vi "CountVectorizer.vi"(8 "error in":errorcluster caption="entrée d'erreur", 11 "CountVectorizer":T1={"encoding"="utf-8", "decode_error"="strict", "strip_accents"="None", "lowercase"=TRUE, "preprocessor"="None", "tokenizer"="None", "stop_words"={"Type"="None", "list"=[]}, "token_pattern"="(?u)\\b\\w\\w+\\b", "ngram_range"={"min_n"=1, "max_n"=1}, "analyzer"="word", "max_df"=1.0, "min_df"=1.0, "max_features"=-1, "vocabulary"={"Clé"=["None"], "Valeur"=[]}, "binary"=FALSE, "dtype"="int"} {"max_features" min=-1; "min_df" min=0.0 max=1.0; "max_df" min=0.0 max=1.0}) -> (0 "error out":errorcluster caption="sortie d'erreur", 3 "CountVectorizer.lvclass":refnum<class "CountVectorizer.lvclass">)   [LabVIEW 2020]
doc: "Convert a collection of text documents to a matrix of token counts\n\nThis implementation produces a sparse representation of the counts using scipy.sparse.csr_matrix.\n\nIf you do not provide an a-priori dictionary and you do not use an analyzer that does some kind of feature selection then the number of features will be equal to the vocabulary size found by analyzing the data.\n\n\nParameters :\n\n- encoding : string, default=’utf-8’\nIf bytes or files are given to analyze, this encoding is used to decode.\n\n- decode_error : {‘strict’, ‘ignore’, ‘replace’}, default=’strict’\nInstruction on what to do if a byte sequence is given to analyze that contains characters not of the given encoding. By default, it is ‘strict’, meaning that a UnicodeDecodeError will be raised. Other values are ‘ignore’ and ‘replace’.\n\n- strip_accents : {‘ascii’, ‘unicode’}, default=None\nRemove accents and perform other character normalization during the preprocessing step. ‘ascii’ is a fast method that only works on characters that have an direct ASCII mapping. ‘unicode’ is a slightly slower method that works on any characters. None (default) does nothing.\n\n- lowercase : bool, default=True\nConvert all characters to lowercase before tokenizing.\n\n- preprocessor : callable, default=None\nOverride the preprocessing (string transformation) stage while preserving the tokenizing and n-grams generation steps. Only applies if analyzer is not callable.\n\n- tokenizer : callable, default=None\nOverride the string tokenization step while preserving the preprocessing and n-grams generation steps. Only applies if analyzer == 'word'.\n\n- stop_words : string {‘english’}, list, default=None\nIf ‘english’, a built-in stop word list for English is used. There are several known issues with ‘english’ and you should consider an alternative.\n\nIf a list, that list is assumed to contain stop words, all of which will be removed from the resulting tokens. Only applies if analyzer == 'word'.\n\nIf None, no stop words will be used. max_df can be set to a value in the range [0.7, 1.0) to automatically detect and filter stop words based on intra corpus document frequency of terms.\n\n- token_pattern : string\nRegular expression denoting what constitutes a “token”, only used if analyzer == 'word'. The default regexp select tokens of 2 or more alphanumeric characters (punctuation is completely ignored and always treated as a token separator).\n\n- ngram_range : tuple (min_n, max_n), default=(1, 1)\nThe lower and upper boundary of the range of n-values for different word n-grams or char n-grams to be extracted. All values of n such such that min_n <= n <= max_n will be used. For example an ngram_range of (1, 1) means only unigrams, (1, 2) means unigrams and bigrams, and (2, 2) means only bigrams. Only applies if analyzer is not callable.\n\n- analyzer : string, {‘word’, ‘char’, ‘char_wb’} or callable, default=’word’\nWhether the feature should be made of word n-gram or character n-grams. Option ‘char_wb’ creates character n-grams only from text inside word boundaries; n-grams at the edges of words are padded with space.\n\nIf a callable is passed it is used to extract the sequence of features out of the raw, unprocessed input.\n\n- max_df : float in range [0.0, 1.0] or int, default=1.0\nWhen building the vocabulary ignore terms that have a document frequency strictly higher than the given threshold (corpus-specific stop words). If float, the parameter represents a proportion of documents, integer absolute counts. This parameter is ignored if vocabulary is not None.\n\n- min_df : float in range [0.0, 1.0] or int, default=1\nWhen building the vocabulary ignore terms that have a document frequency strictly lower than the given threshold. This value is also called cut-off in the literature. If float, the parameter represents a proportion of documents, integer absolute counts. This parameter is ignored if vocabulary is not None.\n\n- max_features : int, default=None=-1\nIf not None, build a vocabulary that only consider the top max_features ordered by term frequency across the corpus.\n\nThis parameter is ignored if vocabulary is not None.\n\n- vocabulary : Mapping or iterable, default=None\nEither a Mapping (e.g., a dict) where keys are terms and values are indices in the feature matrix, or an iterable over terms. If not given, a vocabulary is determined from the input documents. Indices in the mapping should not be repeated and should not have any gap between 0 and the largest index.\n\n- binary : bool, default=False\nIf True, all non zero counts are set to 1. This is useful for discrete probabilistic models that model binary events rather than integer counts.\n\n- dtype : type, default=np.int64\nType of the matrix returned by fit_transform() or transform().\n\n\n\n\nMethods : \n\n- Decode the input into a string of unicode symbols. The decoding strategy depends on the vectorizer parameters.\n\nParameters : doc : str\n The string to decode.\n\nReturns : doc : str\n A string of unicode symbols.\n\n\n- Fit : Learn a vocabulary dictionary of all tokens in the raw documents.\n\nParameters : raw_documents : iterable\n An iterable which yields either str, unicode or file objects.\n\nReturns : String : OK\n\n- Fit Transform : Learn the vocabulary dictionary and return document-term matrix. This is equivalent to fit followed by transform, but more efficiently implemented.\n\nParameters : raw_documents : iterable\n An iterable which yields either str, unicode or file objects.\n\nReturns : X : array of shape (n_samples, n_features)\n Document-term matrix.\n\n- Get Feature Names : Array mapping from feature integer indices to feature name.\n\nReturns : feature_names : list\n A list of feature names.\n\n-Transform : Transform documents to document-term matrix. Extract token counts out of raw text documents using the vocabulary fitted with fit or the one provided to the constructor.\n\nParameters : raw_documents : iterable\n An iterable which yields either str, unicode or file objects.\n\nReturns : X : sparse matrix of shape (n_samples, n_features)\n Document-term matrix."
uses:
  CountVectorizer.lvclass
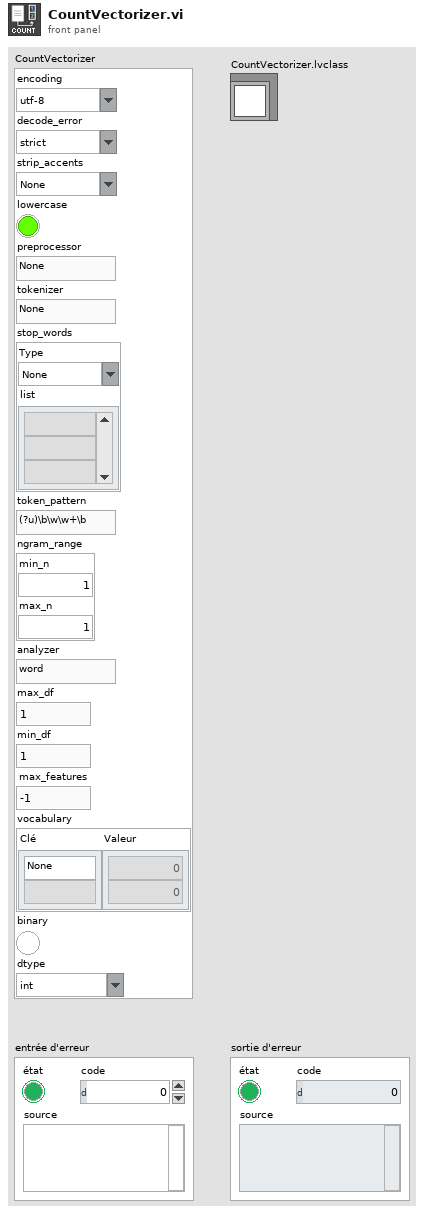
[diagram p1: front panel]
types:
  T1 = cluster{"encoding":string, "decode_error":string, "strip_accents":string, "lowercase":bool, "preprocessor":string, "tokenizer":string, "stop_words":cluster{"Type":string, "list":string[]}, "token_pattern":string, "ngram_range":cluster{"min_n":i32, "max_n":i32}, "analyzer":string, "max_df":dbl, "min_df":dbl, "max_features":i32, "vocabulary":cluster{"Clé":string[], "Valeur":i32[]}, "binary":bool, "dtype":string}
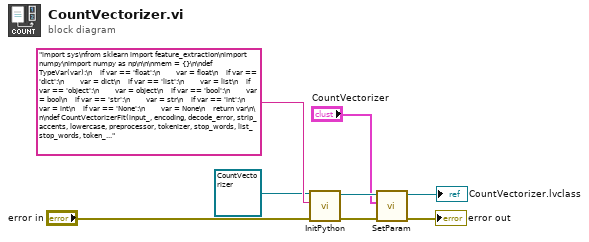
[diagram p0: block diagram]
diagram:
  n1 = call-dynamic "InitPython.vi"("error in (no error)"="error in", "Python Instruction"="import sys\nfrom sklearn import feature_extraction\nimport numpy\nimport numpy as np\n\n\nmem = {}\n\ndef TypeVar(var):\n    if var == 'float':\n        var = float\n    if var == 'dict':\n        var = dict\n    if var == 'list':\n        var = list\n    if var == 'object':\n        var = object\n    if var == 'bool':\n        var = bool\n    if var == 'str':\n        var = str\n    if var == 'int':\n        var = int\n    if var == 'None':\n        var = None\n    return var\n\n\ndef CountVectorizerFit(input_, encoding, decode_error, strip_accents, lowercase, preprocessor, tokenizer, stop_words, list_stop_words, token_pattern, min_n, max_n, analyzer, max_df, min_df, max_features, vocabulary, binary, dtype, X, doc):\n    X = eval(X)\n    dtype = TypeVar(dtype)\n    list_analyzer = ['word', 'char', 'char_wb']\n    if vocabulary == 'None':\n        vocabulary = None\n    else:\n        vocabulary = eval(vocabulary)\n    if tokenizer == 'None' or tokenizer == '':\n        tokenizer = None\n    else:\n        tokenizer = eval(tokenizer)\n    if preprocessor == 'None' or preprocessor == '':\n        preprocessor = None\n    else:\n        preprocessor = eval(preprocessor)\n    if strip_accents == 'None':\n        strip_accents = None\n    if stop_words == 'None':\n        stop_words = None\n    elif stop_words == 'list':\n        stop_words = list_stop_words\n    else: \n        pass\n    if max_features == -1:\n        max_features = None\n    if analyzer not in list_analyzer:\n        analyzer = eval(analyzer)  \n    try:\n        CountVectorizer = feature_extraction.text.CountVectorizer(input_, encoding, decode_error, strip_accents, lowercase, preprocessor, tokenizer, stop_words, token_pattern, (min_n, max_n), analyzer, max_df, min_df, max_features, vocabulary, binary, dtype).fit(X)\n        mem['FitCountVectorizer'] = CountVectorizer\n        return str('OK')\n    except:\n        erreur = sys.exc_info()\n        typerr = u\"%s\" % (erreur[0])\n        typerr = typerr[typerr.find(\"'\")+1:typerr.rfind(\"'\")]\n        msgerr = u\"%s\" % (erreur[1])\n        message = str('/!\\\\ {0} : {1}'. format(typerr,msgerr))\n        return message \n\ndef CountVectorizerFitTransform(input_, encoding, decode_error, strip_accents, lowercase, preprocessor, tokenizer, stop_words, list_stop_words, token_pattern, min_n, max_n, analyzer, max_df, min_df, max_features, vocabulary, binary, dtype, X, doc):\n    X = eval(X)\n    dtype = TypeVar(dtype)\n    list_analyzer = ['word', 'char', 'char_wb']\n    if vocabulary == 'None':\n        vocabulary = None\n    else:\n        vocabulary = eval(vocabulary)\n    if tokenizer == 'None' or tokenizer == '':\n        tokenizer = None\n    else:\n        tokenizer = eval(tokenizer)\n    if preprocessor == 'None' or preprocessor == '':\n        preprocessor = None\n    else:\n        preprocessor = eval(preprocessor)\n    if strip_accents == 'None':\n        strip_accents = None\n    if stop_words == 'None':\n        stop_words = None\n    elif stop_words == 'list':\n        stop_words = list_stop_words\n    else: \n        pass\n    if max_features == -1:\n        max_features = None\n    if analyzer not in list_analyzer:\n        analyzer = eval(analyzer)  \n    try:\n        CountVectorizer = feature_extraction.text.CountVectorizer(input_, encoding, decode_error, strip_accents, lowercase, preprocessor, tokenizer, stop_words, token_pattern, (min_n, max_n), analyzer, max_df, min_df, max_features, vocabulary, binary, dtype).fit_transform(X)\n        dtype = type(CountVectorizer)\n        if dtype == numpy.ndarray:\n            CountVectorizer = CountVectorizer.tolist()\n            return str(CountVectorizer)\n        else:\n            Mat = CountVectorizer.tocoo()\n            return str(list(zip(Mat.row, Mat.col, Mat.data)))\n    except:\n        erreur = sys.exc_info()\n        typerr = u\"%s\" % (erreur[0])\n        typerr = typerr[typerr.find(\"'\")+1:typerr.rfind(\"'\")]\n        msgerr = u\"%s\" % (erreur[1])\n        message = str('/!\\\\ {0} : {1}'. format(typerr,msgerr))\n        return message \n    \ndef CountVectorizerTransform(input_, encoding, decode_error, strip_accents, lowercase, preprocessor, tokenizer, stop_words, list_stop_words, token_pattern, min_n, max_n, analyzer, max_df, min_df, max_features, vocabulary, binary, dtype, X, doc):\n    X = eval(X)\n    dtype = TypeVar(dtype)\n    list_analyzer = ['word', 'char', 'char_wb']\n    if vocabulary == 'None':\n        vocabulary = None\n    else:\n        vocabulary = eval(vocabulary)\n    if tokenizer == 'None' or tokenizer == '':\n        tokenizer = None\n    else:\n        tokenizer = eval(tokenizer)\n    if preprocessor == 'None' or preprocessor == '':\n        preprocessor = None\n    else:\n        preprocessor = eval(preprocessor)\n    if strip_accents == 'None':\n        strip_accents = None\n    if stop_words == 'None':\n        stop_words = None\n    elif stop_words == 'list':\n        stop_words = list_stop_words\n    else: \n        pass\n    if max_features == -1:\n        max_features = None\n    if analyzer not in list_analyzer:\n        analyzer = eval(analyzer)     \n    try:\n        CountVectorizer = mem['FitCountVectorizer'].transform(X)\n        dtype = type(CountVectorizer)\n        if dtype == numpy.ndarray:\n            CountVectorizer = CountVectorizer.tolist()\n            return str(CountVectorizer)\n        else:\n            Mat = CountVectorizer.tocoo()\n            return str(list(zip(Mat.row, Mat.col, Mat.data)))\n    except:\n        erreur = sys.exc_info()\n        typerr = u\"%s\" % (erreur[0])\n        typerr = typerr[typerr.find(\"'\")+1:typerr.rfind(\"'\")]\n        msgerr = u\"%s\" % (erreur[1])\n        message = str('/!\\\\ {0} : {1}'. format(typerr,msgerr))\n        return message\n\ndef CountVectorizerGetFeat(input_, encoding, decode_error, strip_accents, lowercase, preprocessor, tokenizer, stop_words, list_stop_words, token_pattern, min_n, max_n, analyzer, max_df, min_df, max_features, vocabulary, binary, dtype, X, doc):\n    X = eval(X)\n    dtype = TypeVar(dtype)\n    list_analyzer = ['word', 'char', 'char_wb']\n    if vocabulary == 'None':\n        vocabulary = None\n    else:\n        vocabulary = eval(vocabulary)\n    if tokenizer == 'None' or tokenizer == '':\n        tokenizer = None\n    else:\n        tokenizer = eval(tokenizer)\n    if preprocessor == 'None' or preprocessor == '':\n        preprocessor = None\n    else:\n        preprocessor = eval(preprocessor)\n    if strip_accents == 'None':\n        strip_accents = None\n    if stop_words == 'None':\n        stop_words = None\n    elif stop_words == 'list':\n        stop_words = list_stop_words\n    else: \n        pass\n    if max_features == -1:\n        max_features = None\n    if analyzer not in list_analyzer:\n        analyzer = eval(analyzer)    \n    try:\n        CountVectorizer = feature_extraction.text.CountVectorizer(input_, encoding, decode_error, strip_accents, lowercase, preprocessor, tokenizer, stop_words, token_pattern, (min_n, max_n), analyzer, max_df, min_df, max_features, vocabulary, binary, dtype).get_feature_names()\n        return str(CountVectorizer)\n    except:\n        erreur = sys.exc_info()\n        typerr = u\"%s\" % (erreur[0])\n        typerr = typerr[typerr.find(\"'\")+1:typerr.rfind(\"'\")]\n        msgerr = u\"%s\" % (erreur[1])\n        message = str('/!\\\\ {0} : {1}'. format(typerr,msgerr))\n        return message\n    \ndef CountVectorizerDecode(input_, encoding, decode_error, strip_accents, lowercase, preprocessor, tokenizer, stop_words, list_stop_words, token_pattern, min_n, max_n, analyzer, max_df, min_df, max_features, vocabulary, binary, dtype, X, doc):\n    X = eval(X)\n    dtype = TypeVar(dtype)\n    list_analyzer = ['word', 'char', 'char_wb']\n    if vocabulary == 'None':\n        vocabulary = None\n    else:\n        vocabulary = eval(vocabulary)\n    if tokenizer == 'None' or tokenizer == '':\n        tokenizer = None\n    else:\n        tokenizer = eval(tokenizer)\n    if preprocessor == 'None' or preprocessor == '':\n        preprocessor = None\n    else:\n        preprocessor = eval(preprocessor)\n    if strip_accents == 'None':\n        strip_accents = None\n    if stop_words == 'None':\n        stop_words = None\n    elif stop_words == 'list':\n        stop_words = list_stop_words\n    else: \n        pass\n    if max_features == -1:\n        max_features = None\n    if analyzer not in list_analyzer:\n        analyzer = eval(analyzer)   \n    try:\n        CountVectorizer = feature_extraction.text.CountVectorizer(input_, encoding, decode_error, strip_accents, lowercase, preprocessor, tokenizer, stop_words, token_pattern, (min_n, max_n), analyzer, max_df, min_df, max_features, vocabulary, binary, dtype).decode(doc)\n        return str(CountVectorizer)\n    except:\n        erreur = sys.exc_info()\n        typerr = u\"%s\" % (erreur[0])\n        typerr = typerr[typerr.find(\"'\")+1:typerr.rfind(\"'\")]\n        msgerr = u\"%s\" % (erreur[1])\n        message = str('/!\\\\ {0} : {1}'. format(typerr,msgerr))\n        return message", "Scikit-learn en entrée"=refnum<class "CountVectorizer.lvclass"> refnum ("CountVectorizer.lvclass")) -> ("error out"=w5:errorcluster, "Scikit-learn en sortie"=w4:refnum<class "CountVectorizer.lvclass">)  [unwired: 7 in]
  n2 = call-dynamic "SetParam.vi"("error in (no error)"=w5, "CountVectorizer"="CountVectorizer", "CountVectorizer.lvclass"=w4) -> ("error out"=→"error out":errorcluster, "CountVectorizer.lvclass"=→"CountVectorizer.lvclass":refnum<class "CountVectorizer.lvclass">)  [unwired: 7 in]
